vi "Select Resolution.vi"(8 "error in (no error)":errorcluster, 11 "Resolution (nm)":dbl format="%#_13g") -> (0 "error out":errorcluster, 3 "Resolution (6: 1.000nm)":u16(ring)=2 items=["", "0.020nm", "0.050nm", "0.100nm", "0.200nm", "0.500nm", "1.000nm", "2.000nm", "4GHz", "10GHz", "20GHz", "40GHz", "100GHz", "200GHz", "400GHz"])   [LabVIEW 2018, in "Yokogawa AQ6370D.lvlib" / "Yokogawa AQ6370D.lvclass"]
uses:
  Yokogawa AQ6370D.lvclass
panel:
  out "In Range?":bool
  out "x >= y?":bool[](array[boolean])
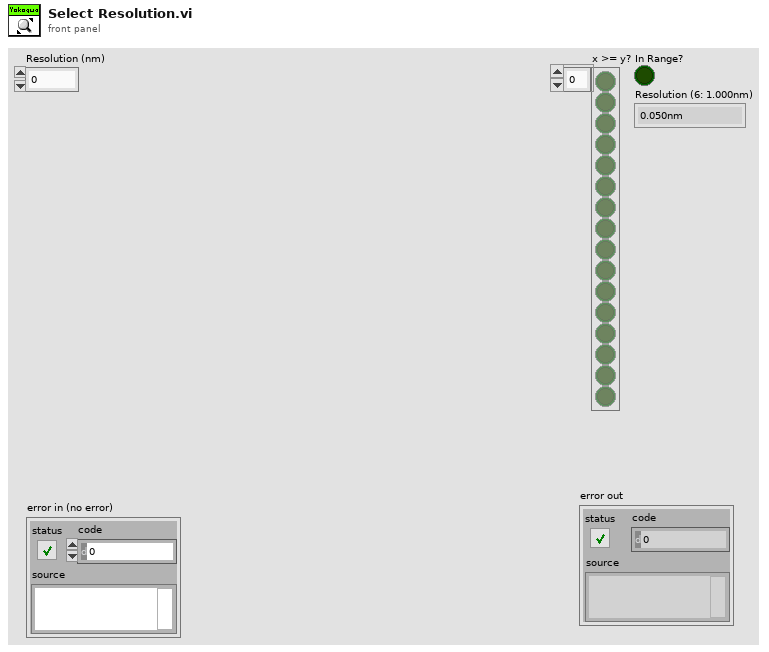
[diagram p1: front panel]
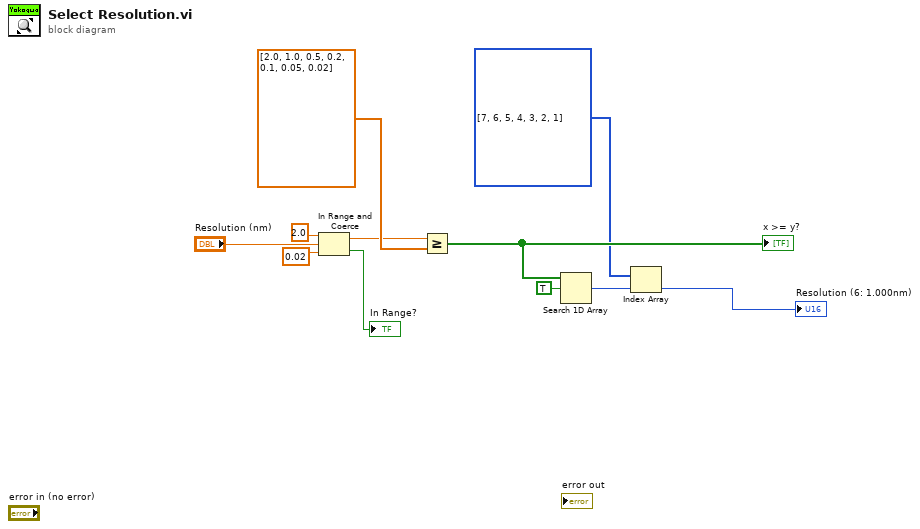
[diagram p0: block diagram]
diagram:
  w3 = u16[] [7, 6, 5, 4, 3, 2, 1] items=["", "0.020nm", "0.050nm", "0.100nm", "0.200nm", "0.500nm", "1.000nm", "2.000nm", "4GHz", "10GHz", "20GHz", "40GHz", "100GHz", "200GHz", "400GHz"]
  n1 = In Range and Coerce(upper limit=2.0, x="Resolution (nm)", lower limit=0.02) -> (coerced(x)=w7:dbl, In Range?=→"In Range?":bool)
  n2 = Greater Or Equal?(x=w7, y=dbl[] [2.0, 1.0, 0.5, 0.2, 0.1, 0.05, 0.02]) -> (x >= y?=w5:bool[])
  "x >= y?" <- w5
  n3 = Search 1D Array(1D array=w5, element=TRUE) -> (index of element=w2:i32)  [unwired: 1 in]
  n4 = Index Array(array=w3, index=w2) -> (element=→"Resolution (6: 1.000nm)":u16)
